vi "Update Card Position.vi"(7 "Card Position Ref":refnum<vi>, 8 "error in (no error)":errorcluster, 9 "NewVal":T2 {"Slot #" max=15}, 10 "OldVal":T2 {"Slot #" max=15}, 11 "Node Ptr in":T1 format="%.0x") -> (0 "error out":errorcluster)   [LabVIEW 2014, in "SLSC configuration System Explorer.lvlib"]
uses:
  SLSC configuration System Explorer.lvlib
  Type Defs/Card Position.ctl
  Shared/SPI Utility/Slot #.ctl
  <vilib>/NI Veristand/Custom Device API/Custom Device Item Ref.ctl
  Shared/Constants.vi
  Shared/SLSC configuration Shared.lvlib
  <vilib>/NI Veristand/Custom Device API/Custom Device API.lvlib
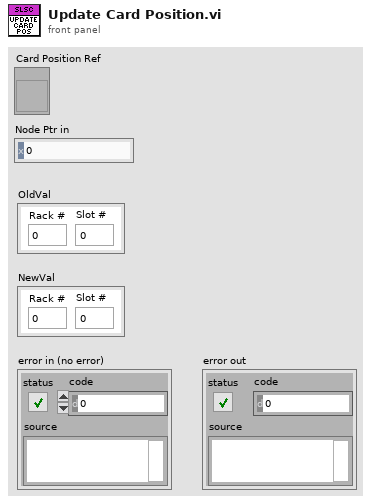
[diagram p1: front panel]
types:
  T1 = typedef "Custom Device API.lvlib/Custom Device Item Ref.ctl" = u64
  T2 = typedef "SLSC configuration Shared.lvlib/Card Position.ctl" = cluster{"Rack #":u8, "Slot #":T3}
  T3 = typedef "SLSC configuration Shared.lvlib/Slot #.ctl" = u8
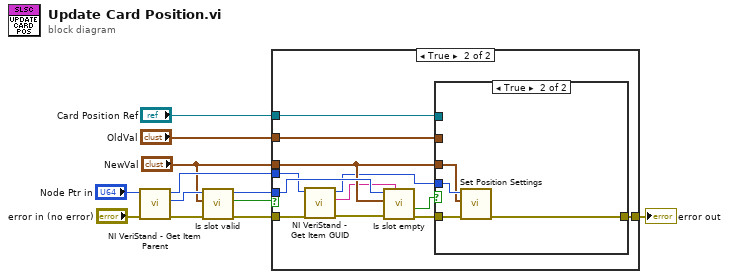
[diagram p0: block diagram]
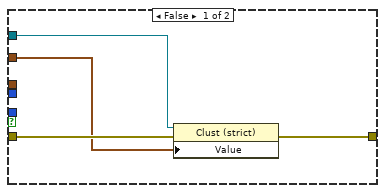
[diagram p2: hidden frame]
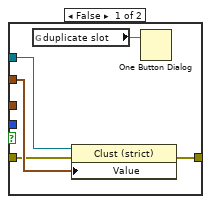
[diagram p3: hidden frame]
diagram:
  n1 = call <vilib>:"NI VeriStand - Get Item Parent.vi"("error in (no error)"="error in (no error)", "Item Ref in"="Node Ptr in") -> ("error out"=w3:errorcluster, "Parent Ref"=w6:T1, "Item Ref out"=w10:T1)  [unwired: 6 in, 1 out]
  n2 = call "Is slot valid.vi"("error in (no error)"=w3, "Card Position"="NewVal", "Device Ref in"=w6) -> ("error out"=w2:errorcluster, "Valid?"=w1:bool, "Device Ref out"=w5:T1)  [unwired: 6 in]
  n3 = case shown="True" w1 {
    tunnel: "OldVal" -> [w13 w28]
    tunnel: w10 -> [_ w20]
    tunnel: [w15 w27] -> w8
    tunnel: "Card Position Ref" -> [w14 w24]
    tunnel: w5 -> [_ w23]
    tunnel: "NewVal" -> [_ w22]
    tunnel: w2 -> [w16 w21]
    frame False {
      n4 = property class="Clust (strict)"(reference=w14, error in=w16, "Value"=w13) -> (error out=w15:errorcluster)  [unwired: 1 out]
    }
    frame True {
      n5 = call <vilib>:"NI VeriStand - Get Item GUID.vi"("error in (no error)"=w21, "Item Ref in"=w20) -> ("error out"=w19:errorcluster, "GUID"=w18:string, "Item Ref out"=w17:T1)  [unwired: 7 in]
      n6 = call "Is slot empty.vi"("Card GUID"=w18, "error in (no error)"=w19, "Card Position"=w22, "Device Ref in"=w23) -> ("error out"=w25:errorcluster, "Empty?"=w26:bool)  [unwired: 5 in, 1 out]
      n7 = case shown="True" w26 {
        tunnel: w25 -> [w30 w37]
        tunnel: [w29 w36] -> w27
        tunnel: w17 -> [_ w35]
        tunnel: w22 -> [_ w34]
        tunnel: w28 -> [w32 _]
        tunnel: w24 -> [w31 _]
        frame False {
          n8 = global read "Constants.vi" "duplicate slot"() -> (w33:string)
          n9 = property class="Clust (strict)"(reference=w31, error in=w30, "Value"=w32) -> (error out=w29:errorcluster)  [unwired: 1 out]
          n10 = One Button Dialog(message=w33) -> ()  [unwired: 1 in, 1 out]
        }
        frame True {
          n11 = call "Set Position Settings.vi"("error in (no error)"=w37, "Card Position"=w34, "Item Ref in"=w35) -> ("error out"=w36:errorcluster)  [unwired: 7 in, 1 out]
        }
      }
    }
  }
  "error out" <- w8
